vi "Test Not In Process Loop When Uninitialized.vi"(8 "error in (no error)":errorcluster, 11 "Test Case In":refnum<class "Process Lifecycle Test.lvclass">) -> (0 "error out":errorcluster, 3 "Test Case Out":refnum<class "Process Lifecycle Test.lvclass">)   [LabVIEW 2020, in "Process Lifecycle Test.lvclass"]
uses:
  Process Lifecycle Test.lvclass
  Process Lifecycle Test.lvclass/Process Lifecycle Test.ctl
  source/Framework/Process/Process.lvclass
  <vilib>/Astemes/LUnit/Test Case.lvclass
  C:/Program Files (x86)/National Instruments/LabVIEW 2020/vi.lib/Astemes/LUnit/Test Case.lvclass
  C:/Program Files (x86)/National Instruments/LabVIEW 2020/vi.lib/Astemes/LUnit/LUnit Runnable.lvclass
  C:/git/astemes-triarc-framework/tests/Lifecycle Test/Process Lifecycle Test.lvclass
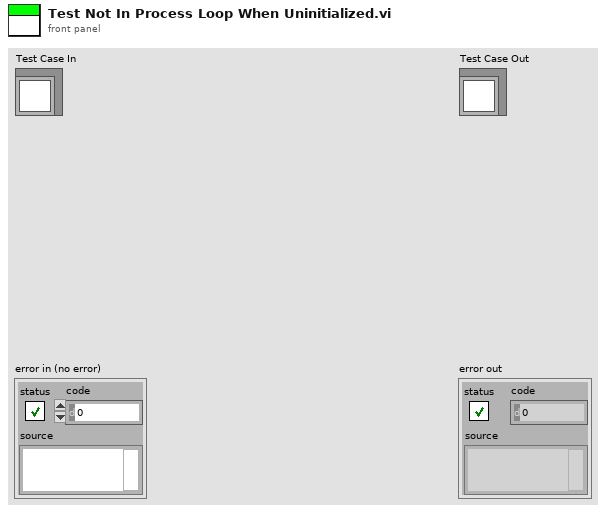
[diagram p1: front panel]
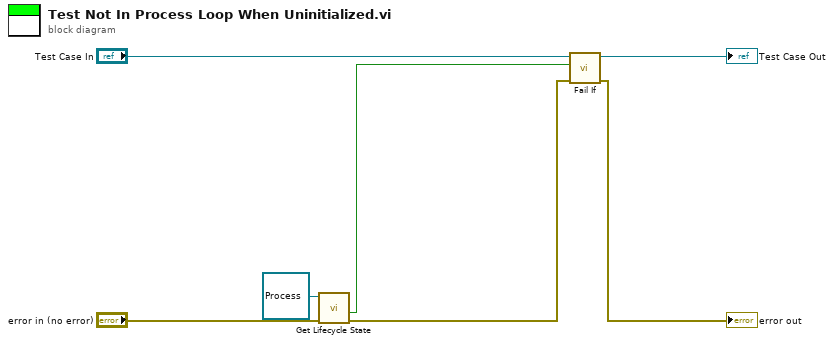
[diagram p0: block diagram]
diagram:
  n1 = call "Get Lifecycle State.vi"("error in (no error)"="error in (no error)", "Process In"=refnum<class "Process.lvclass"> refnum) -> ("error out"=w3:errorcluster, "In Process Loop?"=w1:bool)  [unwired: 6 in, 2 out]
  n2 = call <vilib>:"Fail If.vi"("error in (no error)"=w3, "Fail?"=w1, "LUnit Test Case In"="Test Case In") -> ("error out"=→"error out":errorcluster, "LUnit Test Case Out"=→"Test Case Out":refnum<class "Process Lifecycle Test.lvclass">)  [unwired: 7 in]
